vi "TestRFGVCheckAlarm.vi"() -> (0 "error out":errorcluster, 1 "Alarm 3":bool, 2 "Alarm 2":bool, 3 "Alarm 1":bool)   [LabVIEW 2015]
uses:
  TypeDef/RequestActionEnum.ctl
  LVClasses/Request/PersonnelType.ctl
  TypeDef/PersonnelAndTime.ctl
  TypeDef/Limits.ctl
  LVClasses/Request/Request.lvclass/Request.ctl
  LVClasses/Request/Read Alarm.vi
  LVClasses/Request/Request.lvclass
panel:
  in  "milliseconds to wait":u32
  out "Request":string
  out "Add Request":string
  # "0 FFF"
  # "0, 0, FTF"
  # "300, 500, FFF"
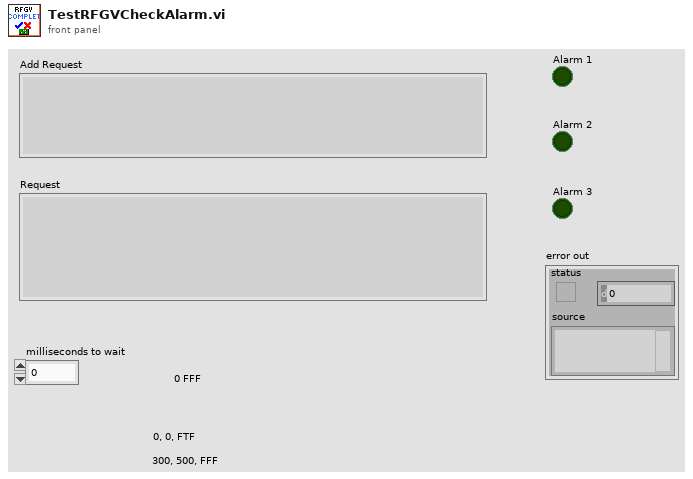
[diagram p1: front panel]
types:
  T1 = typedef "Limits.ctl" = cluster{"AckLimit":dbl, "CompleteLimit":dbl}
  T2 = typedef "RequestActionEnum.ctl" = enum16{"Init", "ReadRequests", "ReadRequest", "AddRequest", "RemoveRequest", "ToDisk", "Ack", "Complete", "CheckAlarms", "PIntoRoom", "Read Summary", "GetRequestForRoom"}
  T3 = typedef "PersonnelAndTime.ctl" = cluster{"Personnel":string, "TimeStamp":string}
  T4 = typedef "Request.lvclass/PersonnelType.ctl" = u16
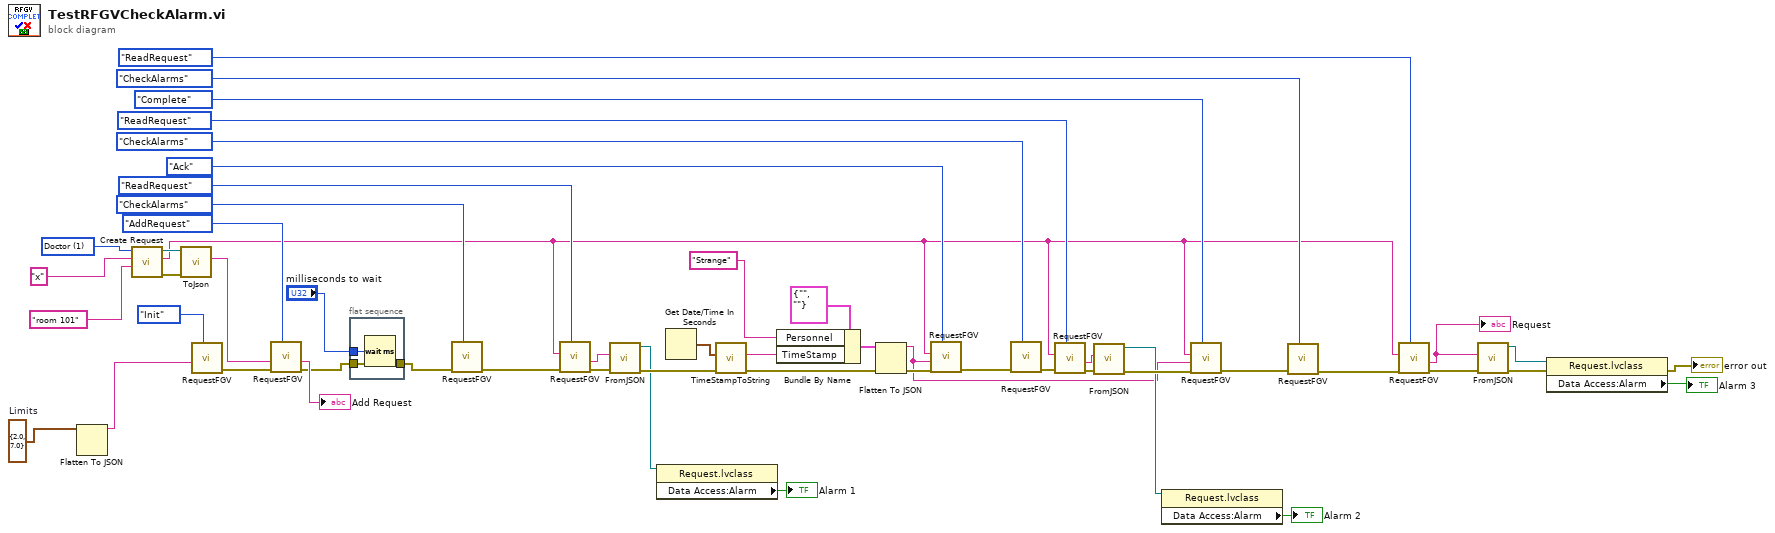
[diagram p0: block diagram]
diagram:
  w2 = T1 {"AckLimit"=2.0, "CompleteLimit"=7.0}  # Limits
  w46 = T4 1 items=["Nurse", "Doctor", "Cleanning", "Admin"] ("Type 2")
  n1 = Flatten To JSON(anything=w2) -> (JSON string=w1:string)  [unwired: 2 in, 1 out]
  n2 = call "Create Request.vi"("Description"="room 101" (".Description 2"), "Name"="x" ("Name 2"), "Personnel Type"=w46) -> ("error out"=w51:errorcluster, "RUID"=w8:string, "Request out"=w50:refnum<class "Request.lvclass">)  [unwired: 6 in]
  n3 = call "ToJson.vi"("error in (no error)"=w51, "Request"=w50) -> ("Request"=w49:string)  [unwired: 8 in, 1 out]
  n4 = call "RequestFGV.vi"("Actions"=RequestActionEnum."Init", "Data In"=w1) -> ("error out"=w43:errorcluster)  [unwired: 8 in, 1 out]
  n5 = call "RequestFGV.vi"("Actions"=RequestActionEnum."AddRequest", "error in (no error)"=w43, "Data In"=w49) -> ("error out"=w7:errorcluster, "Data Out"=→"Add Request":string)  [unwired: 7 in]
  n6 = flat-sequence {
    tunnel: w7 -> [w55]
    tunnel: [w55] -> w6
    tunnel: "milliseconds to wait" -> [w54]
    frame #0 {
      n7 = Wait (ms)(milliseconds to wait=w54) -> ()  [unwired: 1 out]
    }
  }
  n8 = call "RequestFGV.vi"("Actions"=RequestActionEnum."CheckAlarms", "error in (no error)"=w6) -> ("error out"=w28:errorcluster)  [unwired: 8 in, 1 out]
  n9 = call "RequestFGV.vi"("Actions"=RequestActionEnum."ReadRequest", "error in (no error)"=w28, "RUID"=w8) -> ("error out"=w23:errorcluster, "Data Out"=w21:string)  [unwired: 7 in]
  n10 = call "FromJSON.vi"("error in (no error)"=w23, "Request"=w21) -> ("error out"=w22:errorcluster, "Request out"=w20:refnum<class "Request.lvclass">)  [unwired: 8 in]
  n11 = property class="Request.lvclass"(reference=w20) -> ("Data Access:Alarm"=→"Alarm 1":bool)  [unwired: 1 in, 2 out]
  n12 = Get Date/Time In Seconds() -> (seconds since 1Jan1904=w3:timestamp)
  n13 = call "TimeStampToString.vi"("error in (no error)"=w22, "Time Stamp"=w3) -> ("error out"=w39:errorcluster, "String"=w35:string)  [unwired: 8 in]
  n14 = Bundle By Name(cluster=T3 {"Personnel"="", "TimeStamp"=""}, "Personnel"="Strange", "TimeStamp"=w35) -> (w40:T3)
  n15 = Flatten To JSON(anything=w40, error in (no error)=w39) -> (JSON string=w4:string, 11:w26:errorcluster)  [unwired: 1 in]
  n16 = call "RequestFGV.vi"("Actions"=RequestActionEnum."Ack", "error in (no error)"=w26, "Data In"=w4, "RUID"=w8) -> ("error out"=w27:errorcluster)  [unwired: 6 in, 1 out]
  n17 = call "RequestFGV.vi"("Actions"=RequestActionEnum."CheckAlarms", "error in (no error)"=w27) -> ("error out"=w16:errorcluster)  [unwired: 8 in, 1 out]
  n18 = call "RequestFGV.vi"("Actions"=RequestActionEnum."ReadRequest", "error in (no error)"=w16, "RUID"=w8) -> ("error out"=w15:errorcluster, "Data Out"=w14:string)  [unwired: 7 in]
  n19 = call "FromJSON.vi"("error in (no error)"=w15, "Request"=w14) -> ("error out"=w18:errorcluster, "Request out"=w12:refnum<class "Request.lvclass">)  [unwired: 8 in]
  n20 = property class="Request.lvclass"(reference=w12) -> ("Data Access:Alarm"=→"Alarm 2":bool)  [unwired: 1 in, 2 out]
  n21 = call "RequestFGV.vi"("Actions"=RequestActionEnum."Complete", "error in (no error)"=w18, "Data In"=w4, "RUID"=w8) -> ("error out"=w32:errorcluster)  [unwired: 6 in, 1 out]
  n22 = call "RequestFGV.vi"("Actions"=RequestActionEnum."CheckAlarms", "error in (no error)"=w32) -> ("error out"=w31:errorcluster)  [unwired: 8 in, 1 out]
  n23 = call "RequestFGV.vi"("Actions"=RequestActionEnum."ReadRequest", "error in (no error)"=w31, "RUID"=w8) -> ("error out"=w38:errorcluster, "Data Out"=w37:string)  [unwired: 7 in]
  "Request" <- w37
  n24 = call "FromJSON.vi"("error in (no error)"=w38, "Request"=w37) -> ("error out"=w33:errorcluster, "Request out"=w36:refnum<class "Request.lvclass">)  [unwired: 8 in]
  n25 = property class="Request.lvclass"(reference=w36, error in=w33) -> (error out=→"error out":errorcluster, "Data Access:Alarm"=→"Alarm 3":bool)  [unwired: 1 out]
